vi "deinitialize.vi"(0 "HGF_Notifier":refnum<class "HGF_Notifier.lvclass">, 5 "error in (no error)":errorcluster) -> (19 "error out":errorcluster)   [LabVIEW 2014, in "HGF_BaseClasses.lvlib" / "HGF_Notifier.lvclass"]
doc: "This is a dynamic dispatch VI. It can be overwritten by childclasses to release allocated recources."
uses:
  HGF_Notifier.lvclass
  HGF_TriggeredEvent/HGF_TriggeredEvent.lvclass
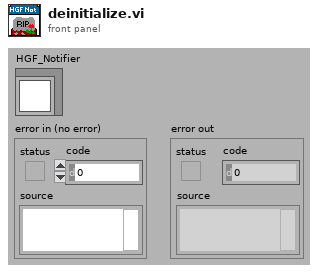
[diagram p1: front panel]
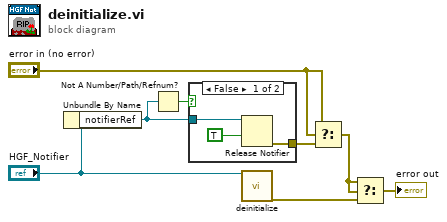
[diagram p0: block diagram]
diagram:
  n1 = Unbundle By Name("HGF_Notifier") -> ("notifierRef"=w2:refnum<notifier>)
  n2 = Not A Number/Path/Refnum?(number/path/refnum=w2) -> (NaN/Path/Refnum?=w1:bool)
  n3 = case shown="False" w1 {
    tunnel: [w11 _] -> w5
    tunnel: w2 -> [w9 _]
    frame False {
      n4 = Release Notifier(notifier=w9, force destroy? (F)=TRUE) -> (error out=w11:errorcluster)  [unwired: 1 in, 2 out]
    }
    frame True {
    }
  }
  n5 = call-parent "deinitialize.vi"("HGF_Factory"="HGF_Notifier") -> ("error out"=w4:errorcluster)  [unwired: 1 in, 17 out]
  n6 = Select(t="error in (no error)", s="error in (no error)", f=w5) -> (s? t:f=w7:errorcluster)
  n7 = Select(t=w7, s=w7, f=w4) -> (s? t:f=→"error out":errorcluster)
